vi "Request-Reply.vi"(8 "error in (no error)":errorcluster, 10 "Number":T1, 11 "API-Reference in":refnum<k1>) -> (0 "error out":errorcluster, 2 "Example Request Out":refnum<k1>, 3 "API-Reference out":refnum<k1>)   [LabVIEW 2018, in "Actor.lvclass"]
uses:
  Actor.lvclass
  API-Data.ctl
  Stopped.ctl
  Event-References.ctl
  Stop.ctl
  Actor Class Launched.ctl
  Example-Request.ctl
  Example-Reply.ctl
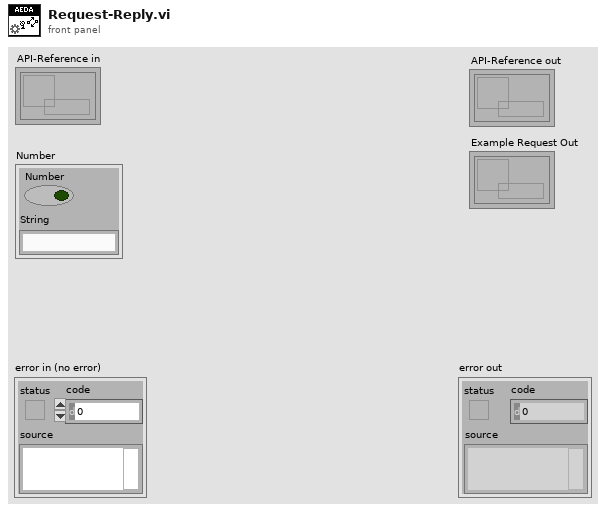
[diagram p1: front panel]
types:
  T1 = typedef "Actor.lvclass/Example-Request.ctl" = cluster{"Number":bool, "String":string}
  T2 = typedef "Actor.lvclass/Example-Reply.ctl" = i32
  T3 = typedef "Actor.lvclass/API-Data.ctl" = cluster{"Launch":refnum<notifier>, "Stopped":refnum<user-event>, "Actor-Events":T4, "Stopped Registration":refnum<event-registration>}
  T4 = typedef "Actor.lvclass/Event-References.ctl" = cluster{"Stop":refnum<user-event>, "Launched":refnum<user-event>, "Example-Request":refnum<user-event>}
  T5 = cluster{"Example-Request":refnum<user-event>, "event data":cluster{"Number":T1, "Reply":refnum<user-event>}}
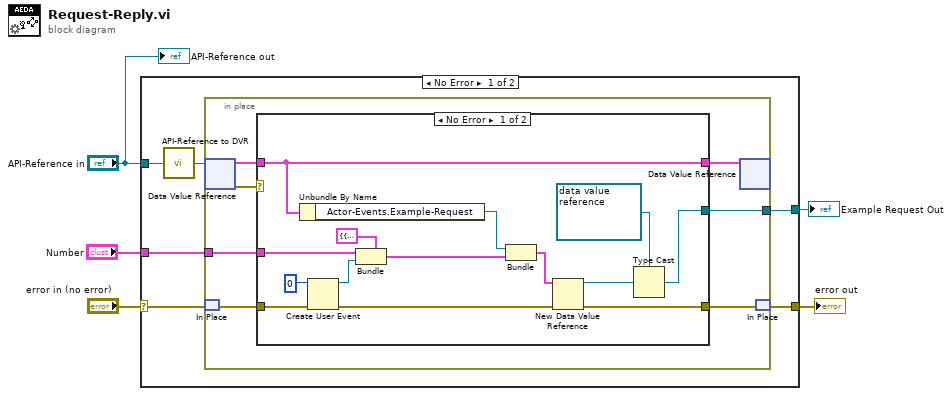
[diagram p0: block diagram]
diagram:
  n1 = case shown="No Error" "error in (no error)" {
    selector: "error in (no error)" -> [w11 w35]
    tunnel: [w10 w35] -> w4
    tunnel: "API-Reference in" -> [w9 _]
    tunnel: "Number" -> [w7 _]
    tunnel: [w6 _] -> w1
    frame No Error {
      n2 = call "API-Reference to DVR.vi"("API-Reference in"=w9) -> ("Data Value Reference out"=w8:refnum<data-value>)
      n3 = in-place {
        in-place-border: w7 -> [w13]
        in-place-border: [w12] -> w6
        n4 = in-place-dvr #1(w8) -> (w17:T3, w18:errorcluster)
        n5 = in-place-match #2(w11) -> (w15:errorcluster)
        n6 = case shown="No Error" w18 {
          selector: w18 -> [_ w34]
          tunnel: w17 -> [w32 w33]
          tunnel: [w32 w33] -> w16
          tunnel: w15 -> [w29 _]
          tunnel: [w22 w34] -> w14
          tunnel: w13 -> [w30 _]
          tunnel: [w19 _] -> w12
          frame No Error {
            n7 = Unbundle By Name(w32) -> ("Actor-Events.Example-Request"=w25:refnum<user-event>)
            n8 = Create User Event(user event datatype=T2 0 ("Result"), error in=w29) -> (user event=w27:refnum<user-event>, error out=w23:errorcluster)
            n9 = Bundle(cluster=cluster{"Number":T1, "Reply":refnum<user-event>} {"Number"={"Number"=FALSE, "String"=""}, "Reply"=refnum} ("event data"), "Number"=w30, "Reply"=w27) -> (w26:cluster{"Number":T1, "Reply":refnum<user-event>})
            n10 = Bundle("Example-Request"=w25, "event data"=w26) -> (w24:T5)  [unwired: 1 in]
            n11 = New Data Value Reference(data value=w24, error in=w23) -> (data value reference=w20:refnum<data-value>, error out=w22:errorcluster)
            n12 = Type Cast(type=refnum<k1> refnum ("API-Reference in"), x=w20) -> (*(type *) &x=w19:refnum<k1>)
          }
          frame Error {
          }
        }
        n13 = in-place-dvr #1(w16) -> ()  [unwired: 2 out]
        n14 = in-place-match #2(w14) -> (w10:errorcluster)
      }
    }
    frame Error {
    }
  }
  "error out" <- w4
  "Example Request Out" <- w1
  "API-Reference out" <- "API-Reference in"
